vi "for自动索引.vi"() -> ()   [LabVIEW 2015]
panel:
  out "Waveform Graph":dbl[](graph)
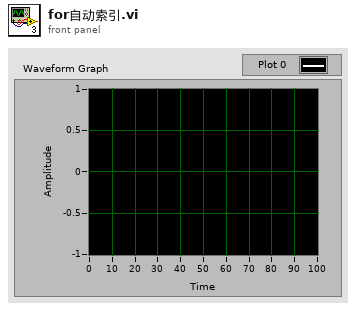
[diagram p1: front panel]
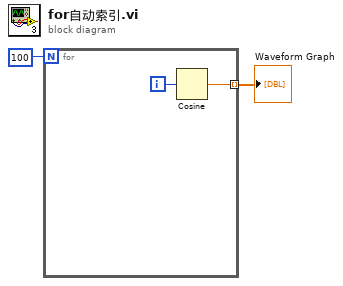
[diagram p0: block diagram]
diagram:
  n1 = for {
    N: 100 -> [_]
    tunnel: [w3] -> w2 mode=indexing
    i -> [w4]
    n2 = Cosine(x=w4) -> (cos(x)=w3:dbl)
  }
  "Waveform Graph" <- w2
